vi "Move File.vi"(8 "error in":errorcluster, 10 "target path":path, 11 "source path":path) -> (0 "error out":errorcluster, 3 "new path":path)   [LabVIEW 2025, in "File System.lvlib"]
uses:
  File System.lvlib
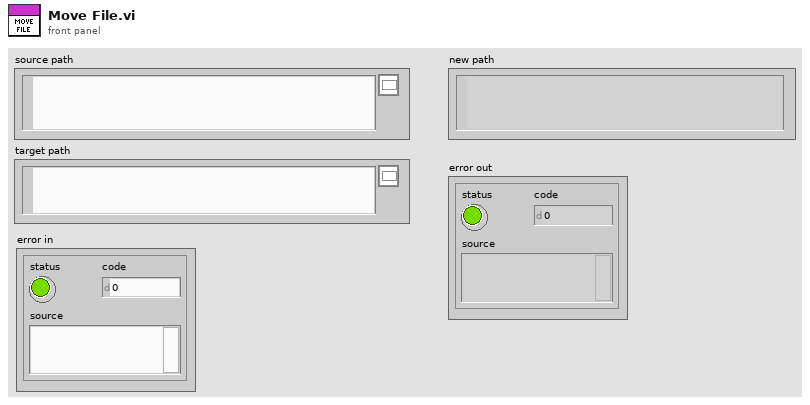
[diagram p1: front panel]
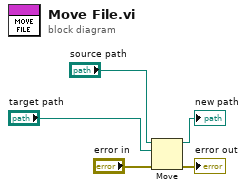
[diagram p0: block diagram]
diagram:
  n1 = Move(source path="source path", error in="error in", 10:"target path") -> (error out=→"error out":errorcluster, 3:→"new path":path)  [unwired: 2 in, 1 out]
